vi "Read DC Power.vi"(8 "error in (no error)":errorcluster, 10 "Platform Slot Number (10)":i16=10 min=-1 max=255, 11 "VISA resource name":refnum<visa-resource-name>) -> (0 "error out":errorcluster, 2 "Power Measurement":dbl format="%#_6e", 3 "VISA resource name out":refnum<visa-resource-name>)   [LabVIEW 2018, in "LTB-1.lvlib" / "3150.lvlib"]
doc: "Reads the power measured at the instrument's input port."
uses:
  3150.lvlib
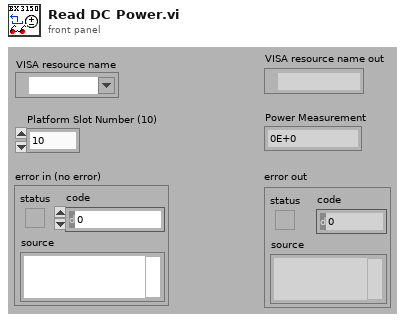
[diagram p1: front panel]
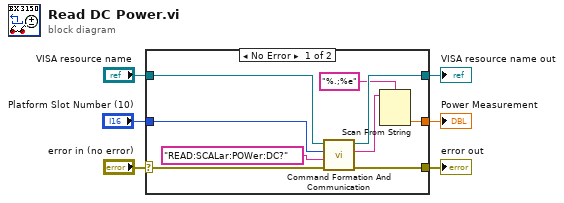
[diagram p0: block diagram]
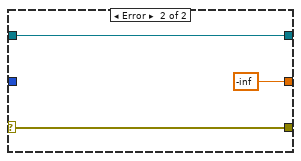
[diagram p2: hidden frame]
diagram:
  n1 = case shown="No Error" "error in (no error)" {
    selector: "error in (no error)" -> [w14 w17]
    tunnel: "VISA resource name" -> [w15 w18]
    tunnel: [w13 w18] -> w4
    tunnel: [w12 w17] -> w3
    tunnel: [w8 -inf] -> w2
    tunnel: "Platform Slot Number (10)" -> [w7 _]
    frame No Error {
      n2 = call "Command Formation And Communication.vi"("error in (no error)"=w14, "Command"="READ:SCALar:POWer:DC?", "Platform Slot Number"=w7, "VISA resource name"=w15) -> ("error out"=w12:errorcluster, "Response"=w9:string, "VISA resource name out"=w13:refnum<visa-resource-name>)  [unwired: 1 in, 4 out]
      n3 = Scan From String(format string="%.;%e", input string=w9) -> (output 1=w8:dbl)  [unwired: 2 in, 4 out]
    }
    frame Error {
    }
  }
  "VISA resource name out" <- w4
  "error out" <- w3
  "Power Measurement" <- w2
